vi "PH_Beckhoff_StepMot.Action Reset.vi"(0 "VI in":refnum<vi>, 5 "error in (no error)":errorcluster) -> (14 "VI out":refnum<vi>, 19 "error out":errorcluster)   [LabVIEW 2014, in "PH_Beckhoff_StepMot.lvlib"]
uses:
  PH_Beckhoff_StepMot.lvlib
  PH_Stepmotor_BaseClass/PH_Stepmotor_BaseClass.lvlib
  non_GPL/instr.lib/Beckhoff/Beckhoff - Driver np.lvlib
  PH_Beckhoff/PH_Beckhoff.lvlib
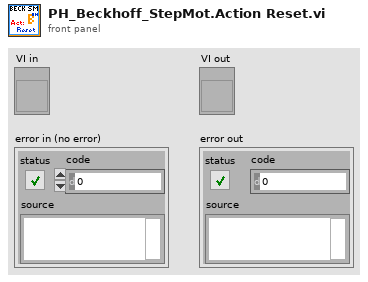
[diagram p1: front panel]
types:
  T1 = typedef "PH_Stepmotor_BaseClass.lvlib/PH_Stepmotor_BaseClass.i attribute.ctl" = cluster{"Device Error":errorcluster, "Axes PSDB Thread":cluster{"Ref":refnum<vi>, "Q-Ref":refnum<queue>, "Data Status":T2}, "Axes":T3[], "Axes PSDB Infos":cluster{"GUI Name":string, "PSDB Instance ID":i32, "PSDB Status Service ID":i32, "Axis":i32, "Class":string}[], "GUI Refs":T8}
  T2 = typedef "PH_PSDBWriter.lvlib/PH_PSDBWriter.Data Status.ctl" = i16
  T3 = typedef "PH_Stepmotor_BaseClass.lvlib/PH_Stepmotor_BaseClass.Axis Attributes.ctl" = cluster{"Settings":T4, "Endswitch?":bool, "DIM Service IDs":T6, "Activity":T7, "Configured?":bool, "Position":cluster{"Current":i32, "Target":i32}, "Position to set":cluster{"New?":bool, "Wanted":i32}, "Stop?":bool, "Reset?":bool, "Move?":bool, "Nothing connected?":bool}
  T4 = typedef "PH_Stepmotor_BaseClass.lvlib/PH_Stepmotor_BaseClass.Axis Settings.ctl" = cluster{"Sign change":bool, "Width":dbl, "Calibration":dbl, "Unit":string, "Motor Type":T5, "Unit Width":string, "Unit CF":string}
  T5 = typedef "PH_Stepmotor_BaseClass.lvlib/PH_Stepmotor_BaseClass.Motor Type.ctl" = enum16{"Unspecific", "OWIS 49.120.2633", "OWIS 49.060.1033", "OWIS 43.040.2558", "Diamond Motion 2200 series", "OWIS 49.120.266B.MV6", "Calorimeter", "Linear Stage 1", "MICOS VT-80", "MICOS VT-80 S", "Standa Rotstage nt0.95A", "PUF RA 320.200", "PUF RA 800.200", "PUF RA 800.400", "PUF RA 400.50", "1324.nn.800.50", "1324.n9c.800.50", "1324.nn.320.200", "1324.nn.400.200", "1324.nn.800.200", "1324.nn.400.50", "1324.8c9c.800.50", "1324.8c9c.400.200"}
  T6 = typedef "PH_Stepmotor_BaseClass.lvlib/PH_Stepmotor_BaseClass.Axis DIM Service IDs.ctl" = cluster{"Settings":i32, "Information":i32}
  T7 = typedef "PH_Stepmotor_BaseClass.lvlib/PH_Stepmotor_BaseClass.Axis Activity.ctl" = enum16{"No Information", "stopped", "running", "Failure", "Alarm", "stopped at backward ES", "stopped at foreward ES"}
  T8 = typedef "PH_Stepmotor_BaseClass.lvlib/PH_Stepmotor_BaseClass.GUI Refs.ctl" = cluster{"Axes Configuration":refnum<vi>, "Device Error":refnum<vi>, "Axes PSDB Infos":refnum<vi>}
  T9 = typedef "PH_Beckhoff.lvlib/PH_Beckhoff.i attribute.ctl" = cluster{"GUI Refs":T10, "operation?":bool, "Default Prdc Interval":i32, "Connection":T11, "AMS Net ID":T12, "Klemmencluster: # of":T13, "Values":T14, "IP":string, "Description":string, "configured?":bool, "Change Manager":cluster{"Detemination wanted?":bool, "Values changed at":cluster{"Sonderklemmen Inputs":i32[], "Analog Inputs":i32[], "Analog Outputs":i32[], "Digital Inputs":i32[], "Digital Outputs":i32[]}}, "Difference to handle an analog input as change":u32}
  T10 = typedef "PH_Beckhoff.lvlib/PH_Beckhoff.GUI Refs.ctl" = cluster{"ADS Error":refnum<vi>, "Values":refnum<vi>, "configured?":refnum<vi>, "Connection":refnum<vi>, "IP":refnum<vi>, "Prdc Int [ms]":refnum<vi>}
  T11 = typedef "PH_Beckhoff.lvlib/PH_Beckhoff.Connectivity.ctl" = cluster{"DLL?":bool, "Port?":bool, "Client?":bool, "Ping?":bool, "unsuccessful Pings":u32}
  T12 = typedef "Beckhoff - Driver np.lvlib/Beckhoff Access.ctl" = cluster{"DLL path":path, "AMS Net ID":cluster{"1st # of IP":u8, "2nd # of IP":u8, "3rd # of IP":u8, "4th # of IP":u8, "In Port":u8, "Out Port":u8}}
  T13 = typedef "Beckhoff - Driver np.lvlib/Klemmendeclarer.ctl" = cluster{"Offset due to Sonderklemms":u32, "analog Inputs":u32, "analog Outputs":u32, "digital Input Bits":u32, "digital Output Bits":u32}
  T14 = typedef "PH_Beckhoff.lvlib/PH_Beckhoff.Values.ctl" = cluster{"Sonderklemmen Inputs":T15, "Analog Inputs":T16, "Analog Outputs":T18, "Digital Inputs":T19, "Digital Outputs":T20}
  T15 = typedef "PH_Beckhoff.lvlib/PH_Beckhoff.Sonderklemmen Inputs.ctl" = cluster{"Total Length":u32, "Name":string, "Value":u64, "Quality":bool, "Service ID":i32, "Offset":u32, "Length":u32}[]
  T16 = typedef "PH_Beckhoff.lvlib/PH_Beckhoff.Analog Inputs.ctl" = cluster{"Name":string, "Value":u32, "Quality":bool, "Service ID":i32, "Sca Type":T17}[]
  T17 = typedef "PH_Beckhoff.lvlib/PH_Beckhoff.Scaling Type.ctl" = enum16{"none", "0 ... 15 Bit -> 0 ... 5", "0 ... 15 Bit -> 0 ... 10", "0 ... 15 Bit -> 0 ... 25", "0 ... 15 Bit -> 4 ... 20", "0 ... 15 Bit -> 0 ... 1", "0 ... 15 Bit -> 0 ... 20000", "0 ... 15 Bit -> 0 ... 24000"}
  T18 = typedef "PH_Beckhoff.lvlib/PH_Beckhoff.Analog Outputs.ctl" = cluster{"Name":string, "Value":u32, "Quality":bool, "Wanted Value":u32, "Service ID":i32, "Sca Type":T17}[]
  T19 = typedef "PH_Beckhoff.lvlib/PH_Beckhoff.Digital Inputs.ctl" = cluster{"Name":string, "Value":bool, "Quality":bool, "Service ID":i32, "inverted?":bool}[]
  T20 = typedef "PH_Beckhoff.lvlib/PH_Beckhoff.Digital Outputs.ctl" = cluster{"Name":string, "Value":bool, "Quality":bool, "Wanted Value":bool, "Service ID":i32, "inverted?":bool}[]
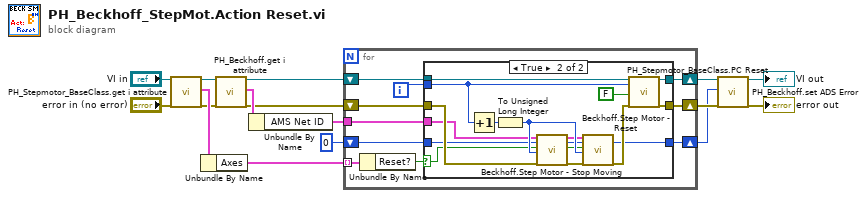
[diagram p0: block diagram]
diagram:
  n1 = call "PH_Stepmotor_BaseClass.get i attribute.vi"("i ref in"="VI in", "error in (no error)"="error in (no error)") -> ("i ref out"=w9:refnum<vi>, "i attribute"=w16:T1, "error out"=w7:errorcluster)  [unwired: 15 in]
  n2 = Unbundle By Name(w16) -> ("Axes"=w15:T3[])
  n3 = call "PH_Beckhoff.get i attribute.vi"("i ref in"=w9, "error in (no error)"=w7) -> ("i ref out"=w8:refnum<vi>, "i attribute"=w14:T9, "error out"=w6:errorcluster)  [unwired: 15 in]
  n4 = Unbundle By Name(w14) -> ("AMS Net ID"=w13:T12)
  n5 = for {
    shift-right: [w25] -> w3
    shift-left: w6 -> [w26]
    shift-right: [w23] -> w5
    shift-left: w8 -> [w24]
    tunnel: w15 -> [w21] mode=indexing
    tunnel: w13 -> [w19]
    shift-right: [w17] -> w1
    shift-left: 0 ("ADS Error in (0)") -> [w18]
    i -> [w22]
    n6 = Unbundle By Name(w21) -> ("Reset?"=w20:bool)
    n7 = case shown="True" w20 {
      selector: w20 -> [_ w32]
      tunnel: w26 -> [w28 w38]
      tunnel: [w28 w46] -> w25
      tunnel: w24 -> [w29 w45]
      tunnel: [w29 w44] -> w23
      tunnel: w22 -> [_ w42]
      tunnel: w19 -> [_ w33]
      tunnel: w18 -> [w27 w31]
      tunnel: [w27 w30] -> w17
      frame False {
      }
      frame True {
        n8 = Increment(x=w42) -> (x+1=w41:i32)
        n9 = To Unsigned Long Integer(number=w41) -> (unsigned 32bit integer=w40:u32)
        n10 = call "Beckhoff.Step Motor - Stop Moving.vi"("AMS Net ID in"=w33, "ADS Error in (0)"=w31, "Write?"=w32, "Klemme"=w40, "error in (no error)"=w38) -> ("AMS Net ID out"=w34:T12, "ADS Error out"=w35:i32, "Write successful?"=w36:bool, "error out"=w39:errorcluster)  [unwired: 11 in]
        n11 = call "Beckhoff.Step Motor - Reset.vi"("AMS Net ID in"=w34, "ADS Error in (0)"=w35, "Write?"=w36, "Klemme"=w40, "error in (no error)"=w39) -> ("ADS Error out"=w30:i32, "error out"=w37:errorcluster)  [unwired: 11 in, 2 out]
        n12 = call "PH_Stepmotor_BaseClass.PC Reset.vi"("i ref in"=w45, "axis"=w42, "Reset?"=FALSE, "error in (no error)"=w37) -> ("i ref out"=w44:refnum<vi>, "error out"=w46:errorcluster)  [unwired: 14 in]
      }
    }
  }
  n13 = call "PH_Beckhoff.set ADS Error.vi"("i ref in"=w5, "ADS Error"=w1, "error in"=w3) -> ("i ref out"=→"VI out":refnum<vi>, "error out"=→"error out":errorcluster)  [unwired: 15 in]
